vi "ImageOperationTest.vi"() -> ()   [LabVIEW 2015]
uses:
  <vilib>/Utility/miscctls.llb/LVRectTypeDef.ctl
  ImageOperation.lvclass
  ImageOperation.lvclass/ImageOperation.ctl
panel:
  in  "SourceFile Path":path
  out "Image":T1(plugin-control)
  in  "Master Bounds Rect":T2
  in  "stop":bool
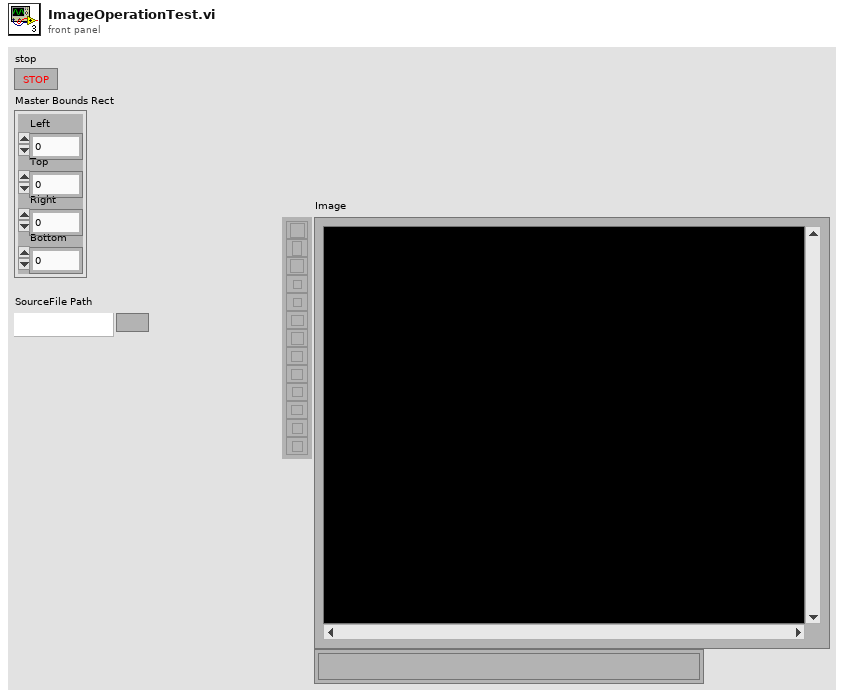
[diagram p1: front panel]
types:
  T1 = typedef "IMAQ Image.ctl" = refnum<image>
  T2 = typedef "LVRectTypeDef.ctl" = cluster{"Left":i16, "Top":i16, "Right":i16, "Bottom":i16}
  T3 = cluster{"Global Rectangle":i32[], "Contours":cluster{"Contour Type":u32, "ROI Type":u32, "Points":i32[]}[]}
  T4 = typedef "Image Type" = u32
  T5 = typedef "ROI Descriptor" = cluster{"Global Rectangle":i32[], "Contours":cluster{"ID":enum32{"External", "Internal"}, "Type":u32, "Coordinates":i32[]}[]}
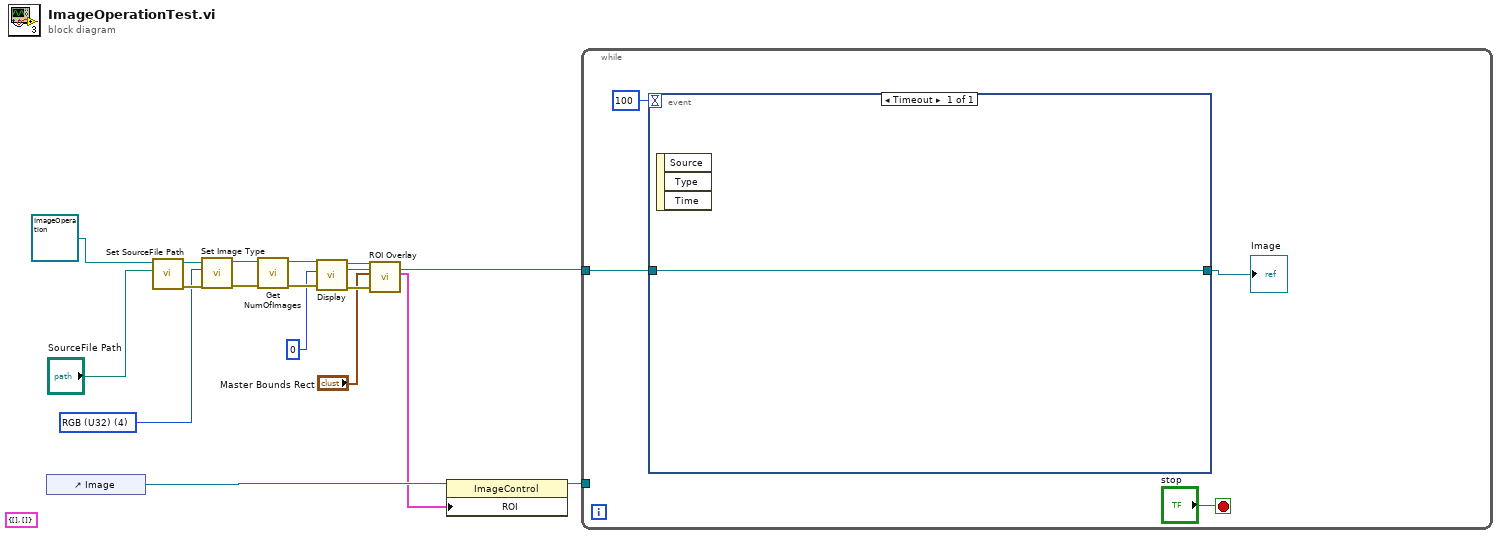
[diagram p0: block diagram]
diagram:
  (unwired) T3 {"Global Rectangle"=[], "Contours"=[]} ("ROI")
  w8 = T4 4 items=["Grayscale (U8)", "Grayscale (I16)", "Grayscale (SGL)", "Complex (CSG)", "RGB (U32)", "HSL (U32)", "RGB (U64)", "Grayscale (U16)"] ("Image Type(U8)")
  n1 = control-ref of="Image"() -> (w6:refnum<vi>)
  n2 = call "Set SourceFile Path.vi"("SourceFile Path"="SourceFile Path", "ImageOperation in"=refnum<class "ImageOperation.lvclass"> refnum ("ImageOperation.lvclass")) -> ("error out"=w11:errorcluster, "ImageOperation out"=w12:refnum<class "ImageOperation.lvclass">)  [unwired: 8 in]
  n3 = call "Set Image Type.vi"("error in (no error)"=w11, "Image Type(U8)"=w8, "ImageOperation in"=w12) -> ("error out"=w9:errorcluster, "ImageOperation out"=w10:refnum<class "ImageOperation.lvclass">)  [unwired: 7 in]
  n4 = call "Get NumOfImages.vi"("error in (no error)"=w9, "ImageOperation in"=w10) -> ("error out"=w15:errorcluster, "ImageOperation out"=w16:refnum<class "ImageOperation.lvclass">)  [unwired: 7 in, 1 out]
  n5 = call "Display.vi"("error in (no error)"=w15, "ImageIndex"=0, "ImageOperation in"=w16) -> ("error out"=w3:errorcluster, "Image Out"=w7:T1, "ImageOperation out"=w4:refnum<class "ImageOperation.lvclass">)  [unwired: 6 in]
  n6 = call "ROI Overlay.vi"("error in (no error)"=w3, "Master Bounds Rect"="Master Bounds Rect", "ImageOperation in"=w4) -> ("ROI Descriptor"=w1:T5)  [unwired: 6 in, 2 out]
  n7 = property class="ImageControl"(reference=w6, "ROI"=w1) -> (reference out=w5:refnum<vi>)  [unwired: 1 in, 1 out]
  n8 = while {
    tunnel: w7 -> [w19]
    tunnel: w5 -> [_]
    stop <- "stop" stop-if-true
    n9 = event shown="[0] Timeout" {
      selector: _ -> [_]
      dyn-events: _ -> [_]
      timeout: 100 -> [_]
      tunnel: w19 -> [w22]
      tunnel: [w22] -> w18
      event Timeout {
        n10 = event-data() -> ()  [unwired: 1 in, 3 out]
      }
    }
    "Image" <- w18
  }
